vi "ArcadeDrive.vi"(0 "FL Wheel Speed":dbl, 1 "BL Wheel Speed":dbl, 2 "FR Wheel Speed":dbl, 3 "BR Wheel Speed":dbl, 4 "FL Wheel Angle":dbl, 5 "BL Wheel Angle":dbl, 6 "FR Wheel Angle":dbl, 7 "BR Wheel Angle":dbl, 10 "ArcadeDrive":bool) -> (20 "New FL Wheel Speed":dbl, 21 "New BL Wheel Speed":dbl, 22 "New FR Wheel Speed":dbl, 23 "New BR Wheel Speed":dbl, 24 "New FL Wheel Angle":dbl, 25 "New BL Wheel Angle":dbl, 26 "New FR Wheel Angle":dbl, 27 "New BR Wheel Angle":dbl)   [LabVIEW 2014]
uses:
  <vilib>/Rock Robotics/WPI/Joystick/WPI_JoystickGetSetRefNum.vi
panel:
  in  "Robot Width":dbl=36.25
  in  "Robot Length":dbl=24.5
  in  "Encoder Offset":dbl
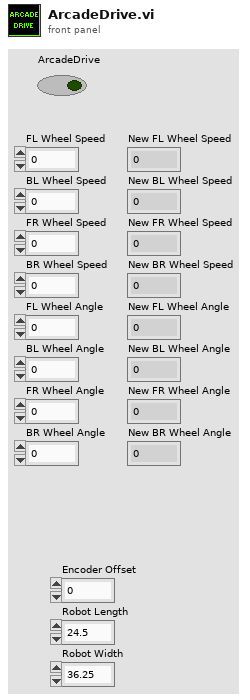
[diagram p1: front panel]
types:
  T1 = typedef "WPI_JoystickDevRef.ctl" = cluster{"Device":T2}
  T2 = typedef "WPI_JoystickDeviceEnum.ctl" = enum16{"USB 0", "USB 1", "USB 2", "USB 3", "USB 4", "USB 5"}
  T3 = typedef "WPI_MotorControlDeviceRef.ctl" = cluster{"DeviceStatus":errorcluster, "Type":T4, "PWM":cluster{"Controller":T5, "PWM Channel":T6, "DeadBand":T7}, "CAN":cluster{"Device Number":u8, "Control Mode":T8, "Semaphore":T9, "Max Vout":dbl, "TalonSRX Control Mode":T10}, "Invert":bool, "TransformRef":T11, "InvTransformRef":T11}
  T4 = typedef "WPI_MotorControlType.ctl" = enum16{"PWM", "CAN", "CANTalonSRX"}
  T5 = typedef "FPGA_TypedefDigitalModule.ctl" = enum16{"Controller 1"}
  T6 = typedef "FPGA_DIOPWMChannel.ctl" = enum8{"PWM 0", "PWM 1", "PWM 2", "PWM 3", "PWM 4", "PWM 5", "PWM 6", "PWM 7", "PWM 8", "PWM 9", "PWM MXP 0", "PWM MXP 1", "PWM MXP 2", "PWM MXP 3", "PWM MXP 4", "PWM MXP 5", "PWM MXP 6", "PWM MXP 7", "PWM MXP 8", "PWM MXP 9", "Invalid"}
  T7 = typedef "WPI_PWMDeadband.ctl" = cluster{"Name":string, "maxPositivePwm":i32, "minPositivePwm":i32, "centerPwm":i32, "maxNegativePwm":i32, "minNegativePwm":i32, "angularRange":u16}
  T8 = typedef "WPI_CANJaguar_ControlMode.ctl" = enum8{"Percent VBus", "Current", "Speed", "Position", "Voltage"}
  T9 = typedef "Semaphore RefNum" = refnum<k1>
  T10 = typedef "WPI_CANTalonSRX_APIControlMode.ctl" = enum8{"Percent VBus", "Speed", "Position", "Slave", "Unchanged / Invalid"}
  T11 = typedef "WPI_PWMTransform_ConPane.ctl" = refnum<vi>
  T12 = typedef "WPI_CANTalonSRX_GlobalStatus.ctl" = cluster{"Applied Throttle":dbl, "Module Enabled":bool, "CAN Error":errorcluster, "Closed Loop Error":dbl, "Forward Limit Switch Closed":bool, "Reverse Limit Switch Closed":bool, "Sensor Position":dbl, "Sensor Velocity":dbl, "Current":dbl, "Sticky Fault - Over Temp":bool, "Sticky Fault - Under Voltage":bool, "Sticky Fault - Forward Limit":bool, "Sticky Fault - Reverse Limit":bool, "Sticky Fault - Forward Soft Limit":bool, "Sticky Fault - Reverse Soft Limit":bool, "Brake is Enabled":bool, "Encoder Position":dbl, "Encoder Velocity":dbl, "Encoder Index Count":dbl, "Encoder A Pin State":bool, "Encoder B Pin State":bool, "Encoder Index Pin State":bool, "Analog In":dbl, "Analog In Velocity":dbl, "Temperature (C)":dbl, "Battery Voltage":dbl}
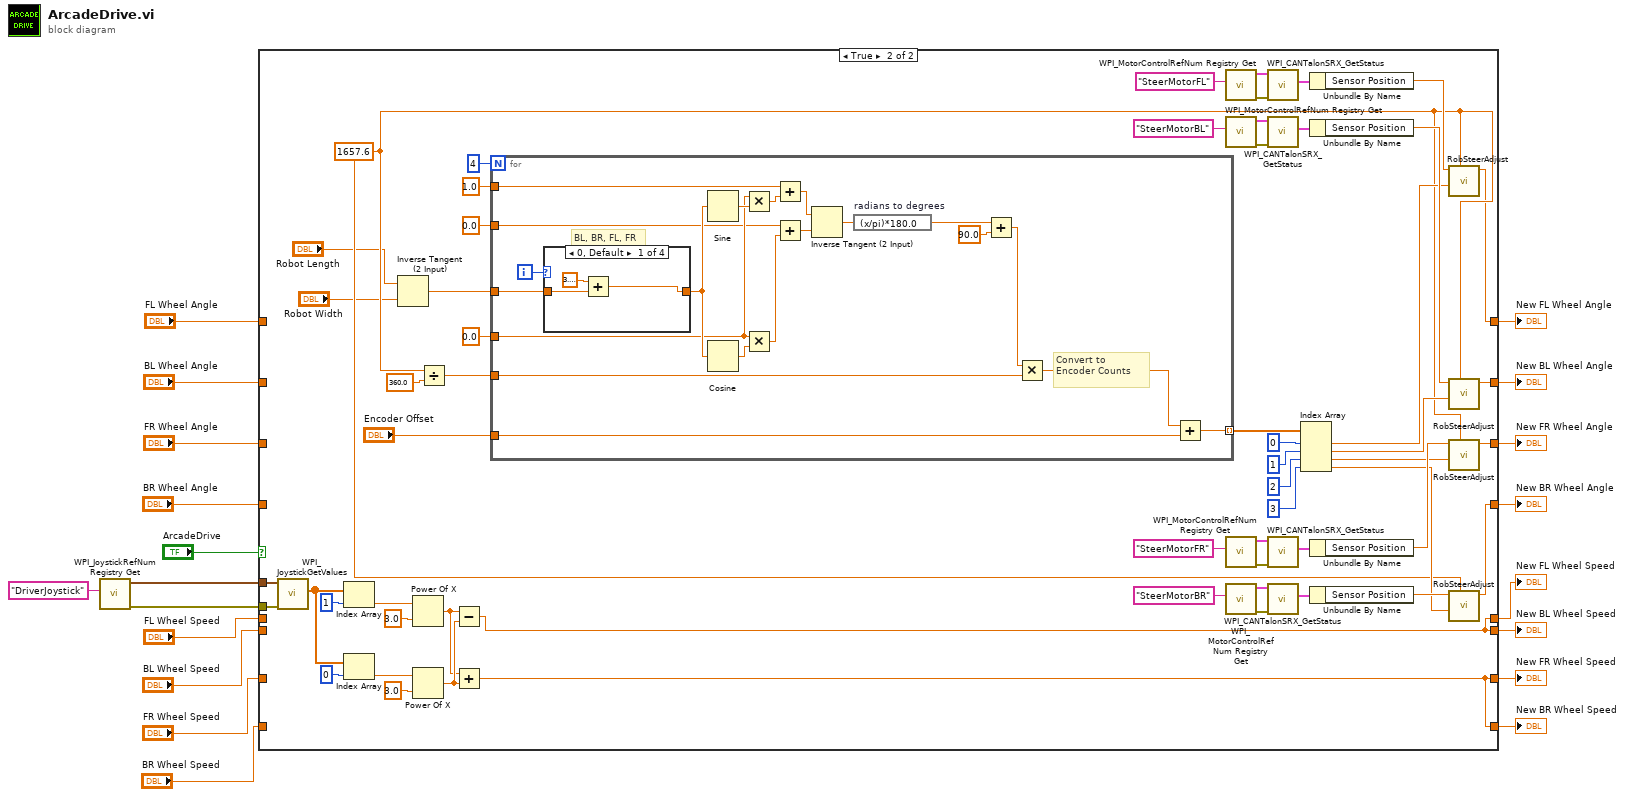
[diagram p0: block diagram]
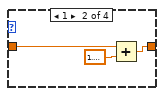
[diagram p3: hidden frame]
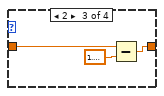
[diagram p4: hidden frame]
diagram:
  n1 = call <vilib>:"WPI_JoystickRefNum Registry Get.vi"("refnum name"="DriverJoystick") -> ("error out"=w17:errorcluster, "JoystickDevRef"=w18:T1)  [unwired: 9 in]
  n2 = case shown="True" "ArcadeDrive" {
    tunnel: w18 -> [_ w85]
    tunnel: w17 -> [_ w84]
    tunnel: "FL Wheel Speed" -> [w28 _]
    tunnel: "BL Wheel Speed" -> [w27 _]
    tunnel: "FR Wheel Speed" -> [w26 _]
    tunnel: "BR Wheel Speed" -> [w25 _]
    tunnel: [w28 w80] -> w12
    tunnel: [w27 w80] -> w11
    tunnel: [w26 w79] -> w10
    tunnel: [w25 w79] -> w9
    tunnel: "FL Wheel Angle" -> [w24 _]
    tunnel: "BL Wheel Angle" -> [w23 _]
    tunnel: "FR Wheel Angle" -> [w22 _]
    tunnel: "BR Wheel Angle" -> [w21 _]
    tunnel: [w24 w38] -> w4
    tunnel: [w23 w37] -> w3
    tunnel: [w22 w36] -> w2
    tunnel: [w21 w35] -> w1
    frame False {
    }
    frame True {
      w70 = 1657.6 ("x")
      n3 = call <vilib>:"WPI_JoystickGetValues.vi"("error in (no error)"=w84, "JoystickDevRef"=w85) -> ("Axes"=w83:dbl[])  [unwired: 5 in, 4 out]
      n4 = Index Array(array=w83, index=1) -> (element=w30:dbl)
      n5 = Index Array(array=w83, index=0) -> (element=w34:dbl)
      n6 = Inverse Tangent (2 Input)(1:"Robot Width", 2:"Robot Length") -> (0:w48:dbl)
      n7 = Power Of X(1:3.0 ("x"), 2:w30) -> (0:w29:dbl)
      n8 = Power Of X(1:3.0 ("x"), 2:w34) -> (0:w32:dbl)
      n9 = Divide(x=w70, y=360.0) -> (x/y=w41:dbl)
      n10 = Subtract(x=w29, y=w32) -> (x-y=w80:dbl)
      n11 = Add(x=w29, y=w32) -> (x+y=w79:dbl)
      n12 = for {
        N: 4 -> [_]
        tunnel: w48 -> [w105]
        tunnel: 0.0 -> [w88]
        tunnel: 0.0 -> [w86]
        tunnel: 1.0 -> [w87]
        tunnel: [w91] -> w49 mode=indexing
        tunnel: w41 -> [w93]
        tunnel: "Encoder Offset" -> [w90]
        i -> [w100]
        # "Convert to\nEncoder Counts"
        # "BL, BR, FL, FR"
        n13 = case shown="0, Default" w100 {
          tunnel: [w107 w111 w114 w115] -> w94
          tunnel: w105 -> [w108 w109 w112 w115]
          frame 0, Default {
            n14 = Add(x=3.141592653589793, y=w108) -> (x+y=w107:dbl)
          }
          frame 1 {
            n15 = Add(x=w109, y=1.5707963267948966) -> (x+y=w111:dbl)
          }
          frame 2 {
            n16 = Subtract(x=w112, y=1.5707963267948966) -> (x-y=w114:dbl)
          }
          frame 3 {
          }
        }
        n17 = Sine(x=w94) -> (sin(x)=w103:dbl)
        n18 = Cosine(x=w94) -> (cos(x)=w104:dbl)
        n19 = Multiply(x=w88, y=w103) -> (x*y=w97:dbl)
        n20 = Multiply(x=w88, y=w104) -> (x*y=w102:dbl)
        n21 = Add(x=w87, y=w97) -> (x+y=w99:dbl)
        n22 = Add(x=w86, y=w102) -> (x+y=w98:dbl)
        n23 = Inverse Tangent (2 Input)(1:w98, 2:w99) -> (0:w101:dbl)
        n24 = expression code="(x/pi)*180.0" "radians to degrees"(w101) -> (w96:dbl)
        n25 = Add(x=w96, y=90.0) -> (x+y=w89:dbl)
        n26 = Multiply(x=w89, y=w93) -> (x*y=w92:dbl)
        n27 = Add(x=w92, y=w90) -> (x+y=w91:dbl)
      }
      n28 = call <vilib>:"WPI_MotorControlRefNum Registry Get.vi"("refnum name"="SteerMotorFL") -> ("error out"=w58:errorcluster, "MotorControlDevRef"=w65:T3)  [unwired: 9 in]
      n29 = call <vilib>:"WPI_MotorControlRefNum Registry Get.vi"("refnum name"="SteerMotorBL") -> ("error out"=w59:errorcluster, "MotorControlDevRef"=w64:T3)  [unwired: 9 in]
      n30 = call <vilib>:"WPI_MotorControlRefNum Registry Get.vi"("refnum name"="SteerMotorFR") -> ("error out"=w60:errorcluster, "MotorControlDevRef"=w63:T3)  [unwired: 9 in]
      n31 = call <vilib>:"WPI_MotorControlRefNum Registry Get.vi"("refnum name"="SteerMotorBR") -> ("error out"=w61:errorcluster, "MotorControlDevRef"=w62:T3)  [unwired: 9 in]
      n32 = call <vilib>:"WPI_CANTalonSRX_GetStatus.vi"("error in (no error)"=w58, "CAN Talon SRX Ref"=w65) -> ("Talon SRX Status"=w66:T12)  [unwired: 7 in, 2 out]
      n33 = call <vilib>:"WPI_CANTalonSRX_GetStatus.vi"("error in (no error)"=w59, "CAN Talon SRX Ref"=w64) -> ("Talon SRX Status"=w67:T12)  [unwired: 7 in, 2 out]
      n34 = call <vilib>:"WPI_CANTalonSRX_GetStatus.vi"("error in (no error)"=w60, "CAN Talon SRX Ref"=w63) -> ("Talon SRX Status"=w68:T12)  [unwired: 7 in, 2 out]
      n35 = call <vilib>:"WPI_CANTalonSRX_GetStatus.vi"("error in (no error)"=w61, "CAN Talon SRX Ref"=w62) -> ("Talon SRX Status"=w69:T12)  [unwired: 7 in, 2 out]
      n36 = Index Array(array=w49, index #1=0 ("index"), index #2=1 ("index"), index #3=2 ("index"), index #4=3 ("index")) -> (element #1=w71:dbl, element #2=w72:dbl, element #3=w73:dbl, element #4=w74:dbl)
      n37 = Unbundle By Name(w66) -> ("Sensor Position"=w75:dbl)
      n38 = Unbundle By Name(w67) -> ("Sensor Position"=w76:dbl)
      n39 = Unbundle By Name(w68) -> ("Sensor Position"=w77:dbl)
      n40 = Unbundle By Name(w69) -> ("Sensor Position"=w78:dbl)
      n41 = call "RobSteerAdjust.vi"("EncoderTicksPerRev"=w70, "Set In"=w71, "Encoder"=w75) -> ("Set Out"=w38:dbl)  [unwired: 8 in]
      n42 = call "RobSteerAdjust.vi"("EncoderTicksPerRev"=w70, "Set In"=w72, "Encoder"=w76) -> ("Set Out"=w37:dbl)  [unwired: 8 in]
      n43 = call "RobSteerAdjust.vi"("EncoderTicksPerRev"=w70, "Set In"=w73, "Encoder"=w77) -> ("Set Out"=w36:dbl)  [unwired: 8 in]
      n44 = call "RobSteerAdjust.vi"("EncoderTicksPerRev"=w70, "Set In"=w74, "Encoder"=w78) -> ("Set Out"=w35:dbl)  [unwired: 8 in]
    }
  }
  "New FL Wheel Speed" <- w12
  "New BL Wheel Speed" <- w11
  "New FR Wheel Speed" <- w10
  "New BR Wheel Speed" <- w9
  "New FL Wheel Angle" <- w4
  "New BL Wheel Angle" <- w3
  "New FR Wheel Angle" <- w2
  "New BR Wheel Angle" <- w1
